vi "re_create_folder.vi"(11 "output folder in":path) -> (3 "output folder out":path)   [LabVIEW 2017]
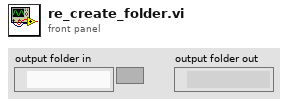
[diagram p1: front panel]
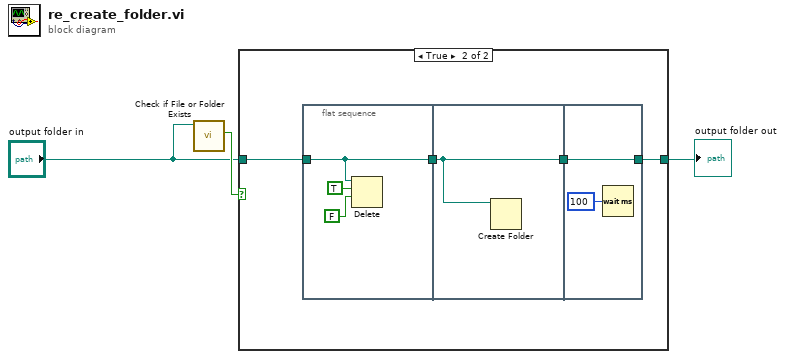
[diagram p0: block diagram]
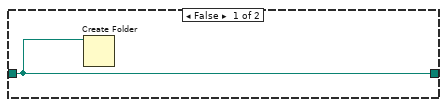
[diagram p2: hidden frame]
diagram:
  n1 = call <vilib>:"Check if File or Folder Exists.vi"("path"="output folder in") -> ("file or folder exists?"=w3:bool)  [unwired: 8 in, 2 out]
  n2 = case shown="True" w3 {
    tunnel: [w4 w7] -> w1
    tunnel: "output folder in" -> [w4 w6]
    frame False {
      n3 = Create Folder(path (use dialog)=w4) -> ()  [unwired: 2 in, 3 out]
    }
    frame True {
      n4 = flat-sequence {
        tunnel: w6 -> [w11]
        tunnel: [w11] -> w8
        tunnel: w8 -> [w12]
        tunnel: [w12] -> w5
        tunnel: [w14] -> w7
        tunnel: w5 -> [w14]
        frame #0 {
          n5 = Delete(path (use dialog)=w11, entire hierarchy (F)=TRUE, confirm (F)=FALSE) -> ()  [unwired: 2 in, 3 out]
        }
        frame #1 {
          n6 = Create Folder(path (use dialog)=w12) -> ()  [unwired: 2 in, 3 out]
        }
        frame #2 {
          n7 = Wait (ms)(milliseconds to wait=u32 100) -> ()  [unwired: 1 out]
        }
      }
    }
  }
  "output folder out" <- w1
